vi "Echo Com Send.vi"(8 "error in (no error)":errorcluster, 9 "Info Data":u16=65535 format="%.0x", 10 "Info Code":u16 format="%.0x", 11 "Port Selection Info":T1={"Port Name"="", "Amplifier Num"=1, "Baud Rate"=38400, "Char Formation"=enum."0"} {"Baud Rate" items=["38400"=38400, "19200"=19200, "9600"=9600, "115200"=0]; "Amplifier Num" max=31}) -> (0 "error out":errorcluster, 1 "Port":refnum<visa-resource-name>, 2 "Bytes Send":u32, 3 "Port Selection Info Out":T1={"Port Name"="", "Amplifier Num"=1, "Baud Rate"=38400, "Char Formation"=enum."0"} {"Baud Rate" items=["38400"=38400, "19200"=19200, "9600"=9600, "115200"=0]; "Amplifier Num" max=31})   [LabVIEW 2014, in "ALPHA5 RS485.lvlib"]
uses:
  ALPHA5 RS485.lvlib
  typedefs/Port Selection Info.ctl
panel:
  # "FC: 08h"
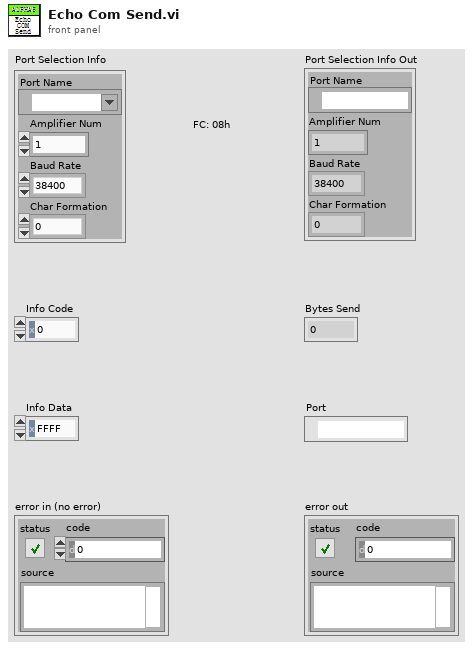
[diagram p1: front panel]
types:
  T1 = typedef "ALPHA5 RS485.lvlib/Port Selection Info.ctl" = cluster{"Port Name":refnum<visa-resource-name>, "Amplifier Num":u8, "Baud Rate":u32, "Char Formation":enum16{"0", "1", "2", "3", "4", "5"}}
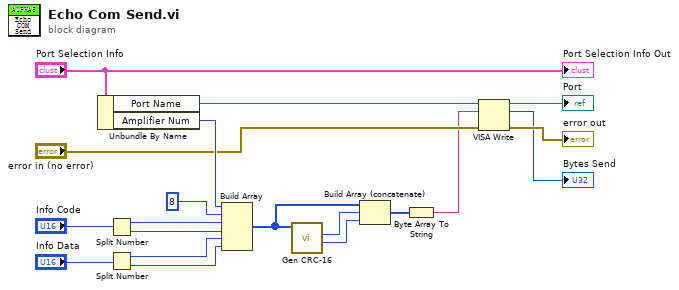
[diagram p0: block diagram]
diagram:
  n1 = Unbundle By Name("Port Selection Info") -> ("Port Name"=w19:refnum<visa-resource-name>, "Amplifier Num"=w18:u8)
  n2 = Split Number(x="Info Code") -> (hi(x)=w14:u8, lo(x)=w13:u8)
  n3 = Split Number(x="Info Data") -> (hi(x)=w12:u8, lo(x)=w11:u8)
  n4 = Build Array(w18, u8 8 ("FC"), w14, w13, w12, w11) -> (w9:u8[])
  n5 = call "Gen CRC-16.vi"("Data In"=w9) -> ("CRC-16-H"=w7:u8, "CRC-16-L"=w8:u8)  [unwired: 7 in, 2 out]
  n6 = Build Array (concatenate)(w9, w8, w7) -> (w6:u8[])
  n7 = Byte Array To String(unsigned byte array=w6) -> (string=w5:string)
  n8 = VISA Write(VISA resource name=w19, write buffer=w5, error in (no error)="error in (no error)") -> (VISA resource name out=→"Port":refnum<visa-resource-name>, return count=→"Bytes Send":u32, error out=→"error out":errorcluster)
  "Port Selection Info Out" <- "Port Selection Info"
